vi "Write Header.vi"(0 "File Path Control":path, 11 "Error In":errorcluster) -> (4 "refnum out":refnum<file>, 6 "File Path":path, 15 "Error Out":errorcluster)   [LabVIEW 2014]
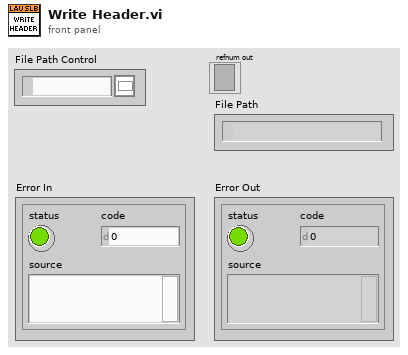
[diagram p1: front panel]
types:
  T1 = enum16{"open", "replace", "create", "open or create", "replace or create", "replace or create with confirmation"}
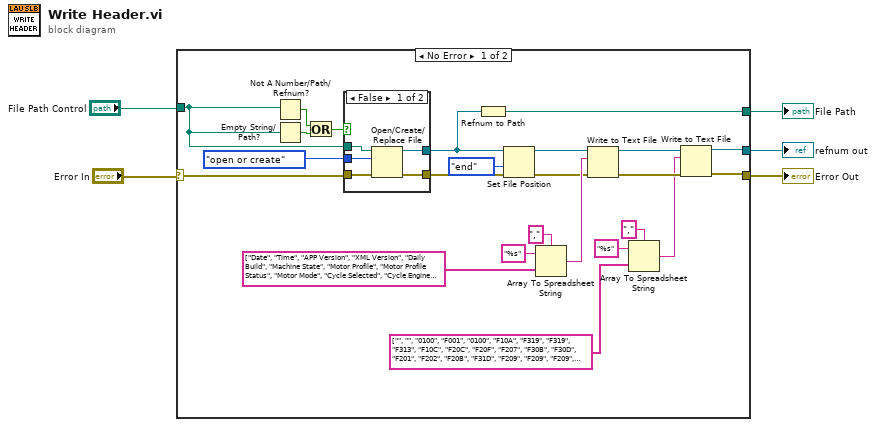
[diagram p0: block diagram]
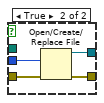
[diagram p2: hidden frame]
diagram:
  n1 = case shown="No Error" "Error In" {
    selector: "Error In" -> [w22 w39]
    tunnel: "File Path Control" -> [w8 _]
    tunnel: [w10 _] -> w4
    tunnel: [w15 w39] -> w2
    tunnel: [w6 _] -> w1
    frame No Error {
      n2 = Not A Number/Path/Refnum?(number/path/refnum=w8) -> (NaN/Path/Refnum?=w26:bool)
      n3 = Empty String/Path?(string/path=w8) -> (empty?=w25:bool)
      n4 = Or(x=w26, y=w25) -> (x .or. y?=w24:bool)
      n5 = case shown="False" w24 {
        tunnel: T1."open or create" ("operation (0:open)") -> [w32 w38]
        tunnel: [w33 w37] -> w7
        tunnel: w8 -> [w34 _]
        tunnel: w22 -> [w31 w36]
        tunnel: [w30 w35] -> w21
        frame False {
          n6 = Open/Create/Replace File(file path (use dialog)=w34, error in=w31, operation (0:open)=w32) -> (refnum out=w33:refnum<file>, error out=w30:errorcluster)  [unwired: 3 in, 1 out]
        }
        frame True {
          n7 = Open/Create/Replace File(error in=w36, operation (0:open)=w38) -> (refnum out=w37:refnum<file>, error out=w35:errorcluster)  [unwired: 4 in, 1 out]
        }
      }
      n8 = Refnum to Path(1:w7) -> (0:w6:path)
      n9 = Set File Position(refnum=w7, from (0:start)=enum16{"start", "end", "current"}."end", error in=w21) -> (refnum out=w18:refnum<file>, error out=w20:errorcluster)  [unwired: 1 in]
      n10 = Array To Spreadsheet String(delimiter (Tab)=",", array=string[] ["Date", "Time", "APP Version", "XML Version", "Daily Build", "Machine State", "Motor Profile", "Motor Profile Status", "Motor Mode", "Cycle Selected", "Cycle Engine Status", "Temperature (F)", "Lid Status", "Basket Speed (RPM)", "Motor Current RMS (AMPS)", "Tub Volume (Gal)", "Pressure (in H2O)", "Lid Lock Status", "Mode Shift Status", "Hot Water Valve", "Cold Water Valve", "Spray/Rinse Valve", "Fabric Softener Valve", "Drain Pump", "Recirculation Pump", "Sub-Cycle", "Cycle Count", "Shaft Speed", "ME Relay", "Valve Relay", "MS Motor", "Deep Fill", "Warm Rinse", "Deep Rinse/FS", "My Cycle", "Extra Rinse", "Temp Level", "Soil Level", "Spin Level", "Load Size", "Stain", "Delay Time", "Soak Time", "Auto Soak Level", "Dry Load Size", "Wet Load Gallons", "Target Gallons", "Load Type", "Target Level (inches)", "Mode Shift Feedback", "Red. Version", "Red. Pressure", "Red. Shaft Speed", "Red. Mode Shift FB", "Red. Lid Switch", "Red. Lid Lock", "Red. Motor Enable", "Red. Triac Enable", "Red. Drain Pump", "Red. Lid Lock  Speed Interlock", "Red. Flood State", "Red. Lid Open  Fault State", "Red. Unlock Fault State", "Red. Access to Moving Parts", "Redundant Heartbeat", "Segment Gallons", "Target Bath Temp (F)", "Current Bath Temp (F)", "ERD 1", "ERD 2", "ERD 3", "Lid Lock FB", "Hot Gallons", "Cold Gallons", "Hot Inlet Temp", "Cold Inlet temp", "Warm Inlet Temp", "Hot Seg Valve Time", "Cold Seg Valve Time", "Coast Time", "Ramp Time", "Ramp Speed", "Ramp Avg Current", "Partial Coast Time", "Dry Load Size", "Ramp Line Voltage", "Coast Line Voltage", "Lid Lock Req State", "OOB Det in Accel", "Folding in Accel", "Max Jerk in Accel", "OOB det in S-S", "Max Jerk in S-S", "OOB Redist Req", "Remaining Cycle Time (s)", "Available Free Stack %", "Child Safety", "Target Speed", "Fault 0", "Fault 1", "Fault 2", "Fault 3", "Fault 4", "Fault 5", "Fault 6", "Fault 7", "Fault 8", "Fault 9", "Personality", "Reset Source"], 3:"%s" ("format string")) -> (spreadsheet string=w27:string)
      n11 = Write to Text File(file (use dialog)=w18, text=w27, error in=w20) -> (refnum out=w11:refnum<file>, error out=w16:errorcluster)  [unwired: 1 in, 1 out]
      n12 = Array To Spreadsheet String(delimiter (Tab)=",", array=string[] ["", "", "0100", "F001", "0100", "F10A", "F319", "F319", "F313", "F10C", "F20C", "F20F", "F207", "F30B", "F30D", "F201", "F202", "F20B", "F31D", "F209", "F209", "F209", "F209", "F210", "F211", "F213", "008E", "F30A", "F321", "F218", "F323", "F123", "F124", "F102", "F103", "F101", "F108", "2015", "F106", "F109", "F107", "2010", "F10E", "F11E", "F305", "F200", "F205", "F206", "F215", "F322", "F011", "F011", "F011", "F011", "F011", "F011", "F011", "F011", "F011", "F011", "F011", "F011", "F011", "F011", "F011", "F22B", "F221", "F222", "ERD 1", "ERD 2", "ERD 3", "F219", "F226", "F226", "F224", "F223", "F225", "F227", "F227", "F304", "F303", "F302", "F300", "F32D", "F305", "F32E", "F301", "F20A", "F315", "F306", "F307", "F316", "F308", "F317", "F140", "F014", "F22A", "F30E", "E064", "E065", "E066", "E067", "E068", "E069", "E06A", "E06B", "E06C", "E06D", "F000", "F017"], 3:"%s" ("format string")) -> (spreadsheet string=w12:string)
      n13 = Write to Text File(file (use dialog)=w11, text=w12, error in=w16) -> (refnum out=w10:refnum<file>, error out=w15:errorcluster)  [unwired: 1 in, 1 out]
    }
    frame Error {
    }
  }
  "Error Out" <- w2
  "refnum out" <- w4
  "File Path" <- w1
